vi "Initialize-UI.vi"(8 "error in (no error)":errorcluster, 10 "Main VI ref":refnum<vi>, 11 "Object ref in":T1) -> (0 "error out":errorcluster, 3 "Object ref out":T1)   [LabVIEW 2013, in "MaterialCharacterization.lvlib" / "MC-Main.lvclass"]
uses:
  MC-Main.lvclass
  Object-reference.ctl
  UI/Pane-settings.ctl
  UI/Pane-names.ctl
  UI/Splitter-settings.ctl
  UI/Splitter-names.ctl
  MC-Main.lvclass/MC-Main.ctl
  UI/MC-UI.lvclass
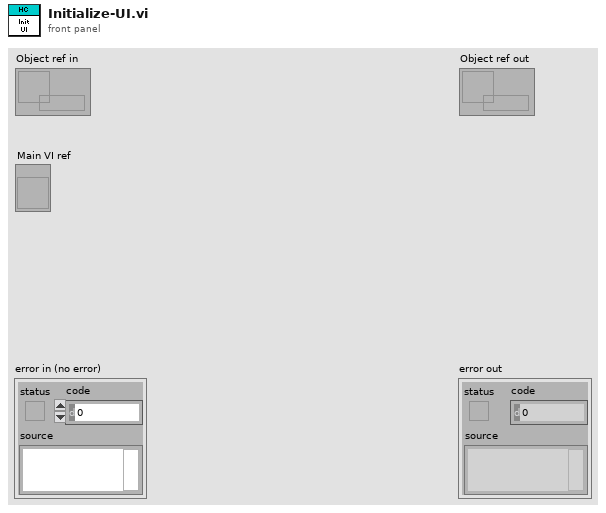
[diagram p1: front panel]
types:
  T1 = typedef "MaterialCharacterization.lvlib/MC-Main.lvclass/Object-reference.ctl" = refnum<data-value>
  T2 = typedef "MaterialCharacterization.lvlib/MC-UI.lvclass/Pane-settings.ctl" = cluster{"Pane-name":T3, "Startup status":bool, "Current status":bool, "Splitters":T4[], "Pane-reference":refnum<vi>}
  T3 = typedef "MaterialCharacterization.lvlib/MC-UI.lvclass/Pane-names.ctl" = enum16{"Toolbar", "Help bar", "Toolbar lower border", "Center panel", "Main panel", "Settings panel", "Status bar upper border", "General state bar", "Information bar"}
  T4 = typedef "MaterialCharacterization.lvlib/MC-UI.lvclass/Splitter-settings.ctl" = cluster{"Splitter-name":T5, "Position shown":i32, "Position hidden":i32, "Splitter reference":refnum<vi>}
  T5 = typedef "MaterialCharacterization.lvlib/MC-UI.lvclass/Splitter-names.ctl" = enum16{"Upper toolbar splitter", "Help bar splitter", "Lower toolbar splitter", "Upper status bar splitter", "Lower status bar splitter", "Left status bar splitter", "Settings splitter"}
  T6 = typedef "MaterialCharacterization.lvlib/MC-UI.lvclass/Panes-reference.ctl" = refnum<data-value>
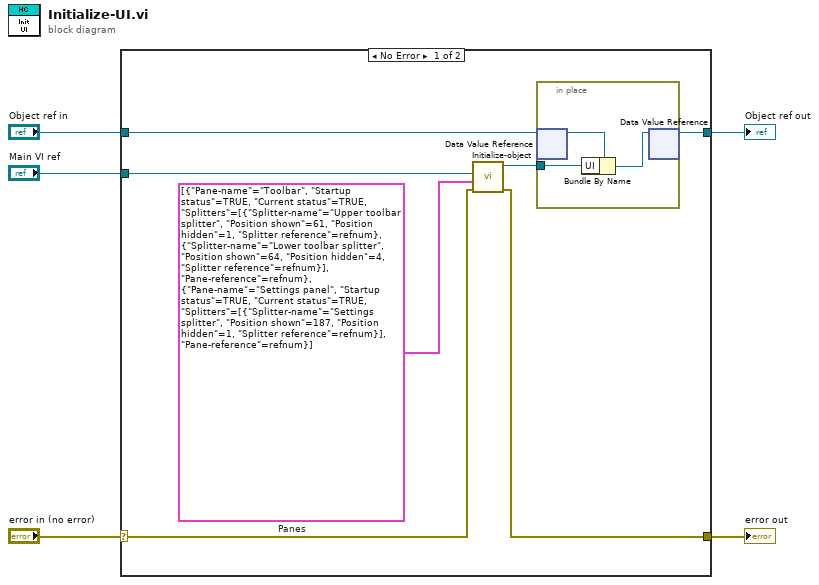
[diagram p0: block diagram]
diagram:
  n1 = case shown="No Error" "error in (no error)" {
    selector: "error in (no error)" -> [w7 w17]
    tunnel: [w8 w17] -> w4
    tunnel: [w11 w16] -> w2
    tunnel: "Object ref in" -> [w12 w16]
    tunnel: "Main VI ref" -> [w9 _]
    frame No Error {
      w6 = T2[] [{"Pane-name"=enum."Toolbar", "Startup status"=TRUE, "Current status"=TRUE, "Splitters"=[{"Splitter-name"=enum."Upper toolbar splitter", "Position shown"=61, "Position hidden"=1, "Splitter reference"=refnum}, {"Splitter-name"=enum."Lower toolbar splitter", "Position shown"=64, "Position hidden"=4, "Splitter reference"=refnum}], "Pane-reference"=refnum}, {"Pane-name"=enum."Settings panel", "Startup status"=TRUE, "Current status"=TRUE, "Splitters"=[{"Splitter-name"=enum."Settings splitter", "Position shown"=187, "Position hidden"=1, "Splitter reference"=refnum}], "Pane-reference"=refnum}]  # Panes
      n2 = call "Initialize-object.vi"("error in (no error)"=w7, "Panes settings"=w6, "VI Reference"=w9) -> ("error out"=w8:errorcluster, "Panes out"=w10:T6)  [unwired: 7 in]
      n3 = in-place {
        in-place-border: w10 -> [w13]
        n4 = in-place-dvr #1(w12) -> (w15:refnum<class "MC-Main.lvclass">)  [unwired: 1 out]
        n5 = Bundle By Name(cluster=w15, "UI"=w13) -> (w14:refnum<class "MC-Main.lvclass">)
        n6 = in-place-dvr #1(w14) -> (w11:T1)  [unwired: 1 out]
      }
    }
    frame Error {
    }
  }
  "error out" <- w4
  "Object ref out" <- w2
